vi "Read Allow Multiple Names.vi"(8 "error in (no error)":errorcluster, 11 "DAQChannelName.lvclass in":refnum<class "DAQChannelName.lvclass">) -> (0 "error out":errorcluster, 2 "AllowMultNames":bool, 3 "DAQChannelName.lvclass out":refnum<class "DAQChannelName.lvclass">)   [LabVIEW 2015, in "DAQChannelName.lvclass"]
uses:
  DAQChannelName.lvclass
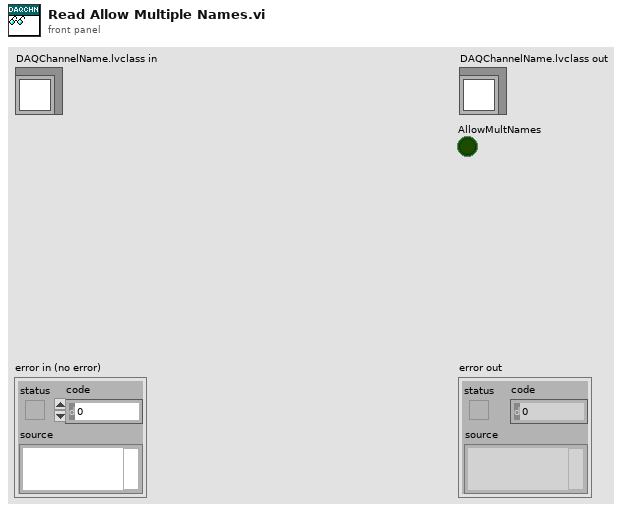
[diagram p1: front panel]
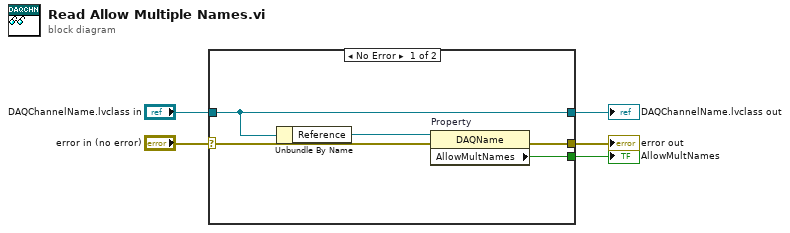
[diagram p0: block diagram]
diagram:
  n1 = case shown="No Error" "error in (no error)" {
    selector: "error in (no error)" -> [w6 w12]
    tunnel: [w9 w12] -> w4
    tunnel: [w8 w11] -> w2
    tunnel: "DAQChannelName.lvclass in" -> [w8 w11]
    tunnel: [w10 _] -> w1
    frame No Error {
      n2 = Unbundle By Name(w8) -> ("Reference"=w7:refnum<vi>)
      n3 = property on="Property" class="DAQName"(reference=w7, error in=w6) -> (error out=w9:errorcluster, "AllowMultNames"=w10:bool)  [unwired: 1 out]
    }
    frame Error {
    }
  }
  "error out" <- w4
  "DAQChannelName.lvclass out" <- w2
  "AllowMultNames" <- w1
